vi "MES字符串.vi"(10 "MES配置输入":T2, 11 "条码字符串输入":T1) -> (2 "MES字符串":string, 3 "2~100":string)   [LabVIEW 2011]
panel:
  out "数组":string[](array[string])
  out "连接的字符串":string
  out "数组 2":string[](array[string])
  out "日期字符串":string
  out "时间字符串":string
  out "56~100":string[](array[string])
  out "已删除元素的数组子集":string[](array[string])
  out "2~55":string
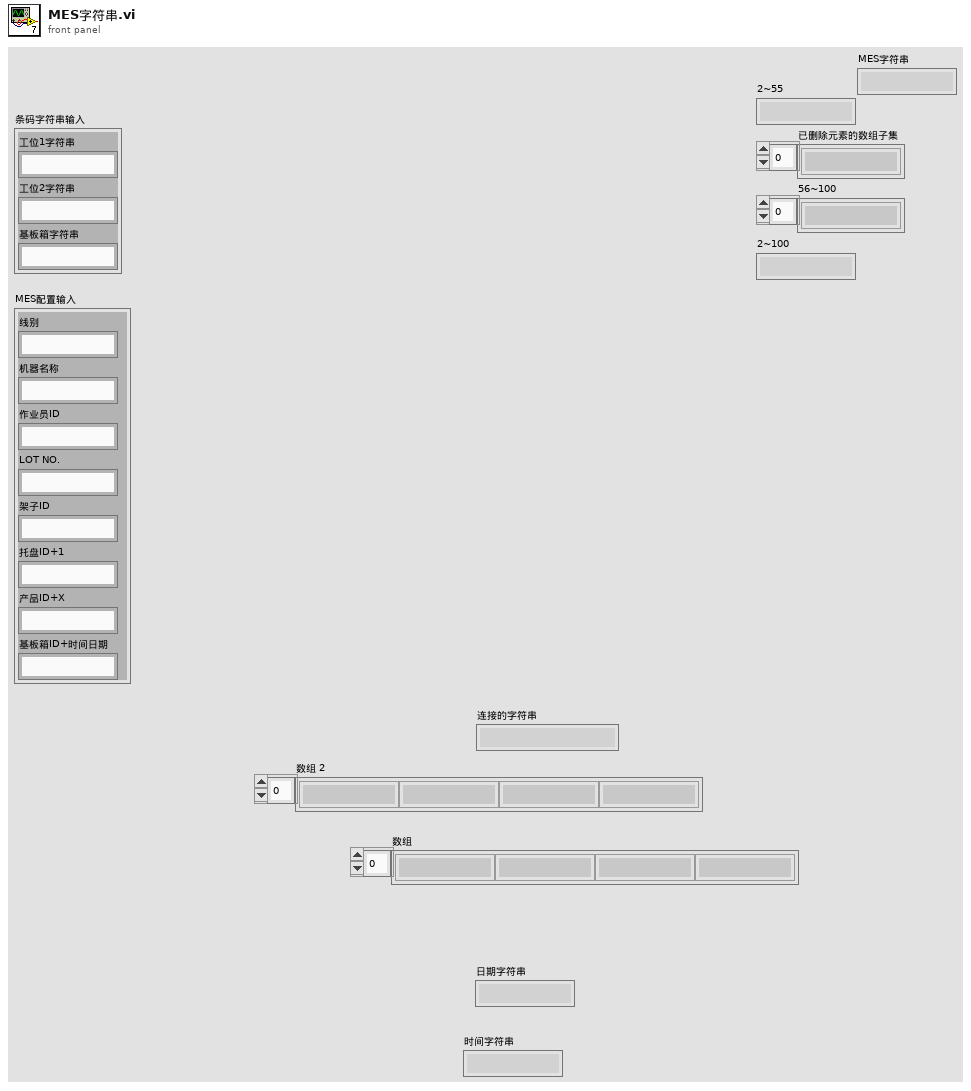
[diagram p1: front panel]
types:
  T1 = cluster{"工位1字符串":string, "工位2字符串":string, "基板箱字符串":string}
  T2 = cluster{"线别":string, "机器名称":string, "作业员ID":string, "LOT NO.":string, "架子ID":string, "托盘ID+1":string, "产品ID+X":string, "基板箱ID+时间日期":string}
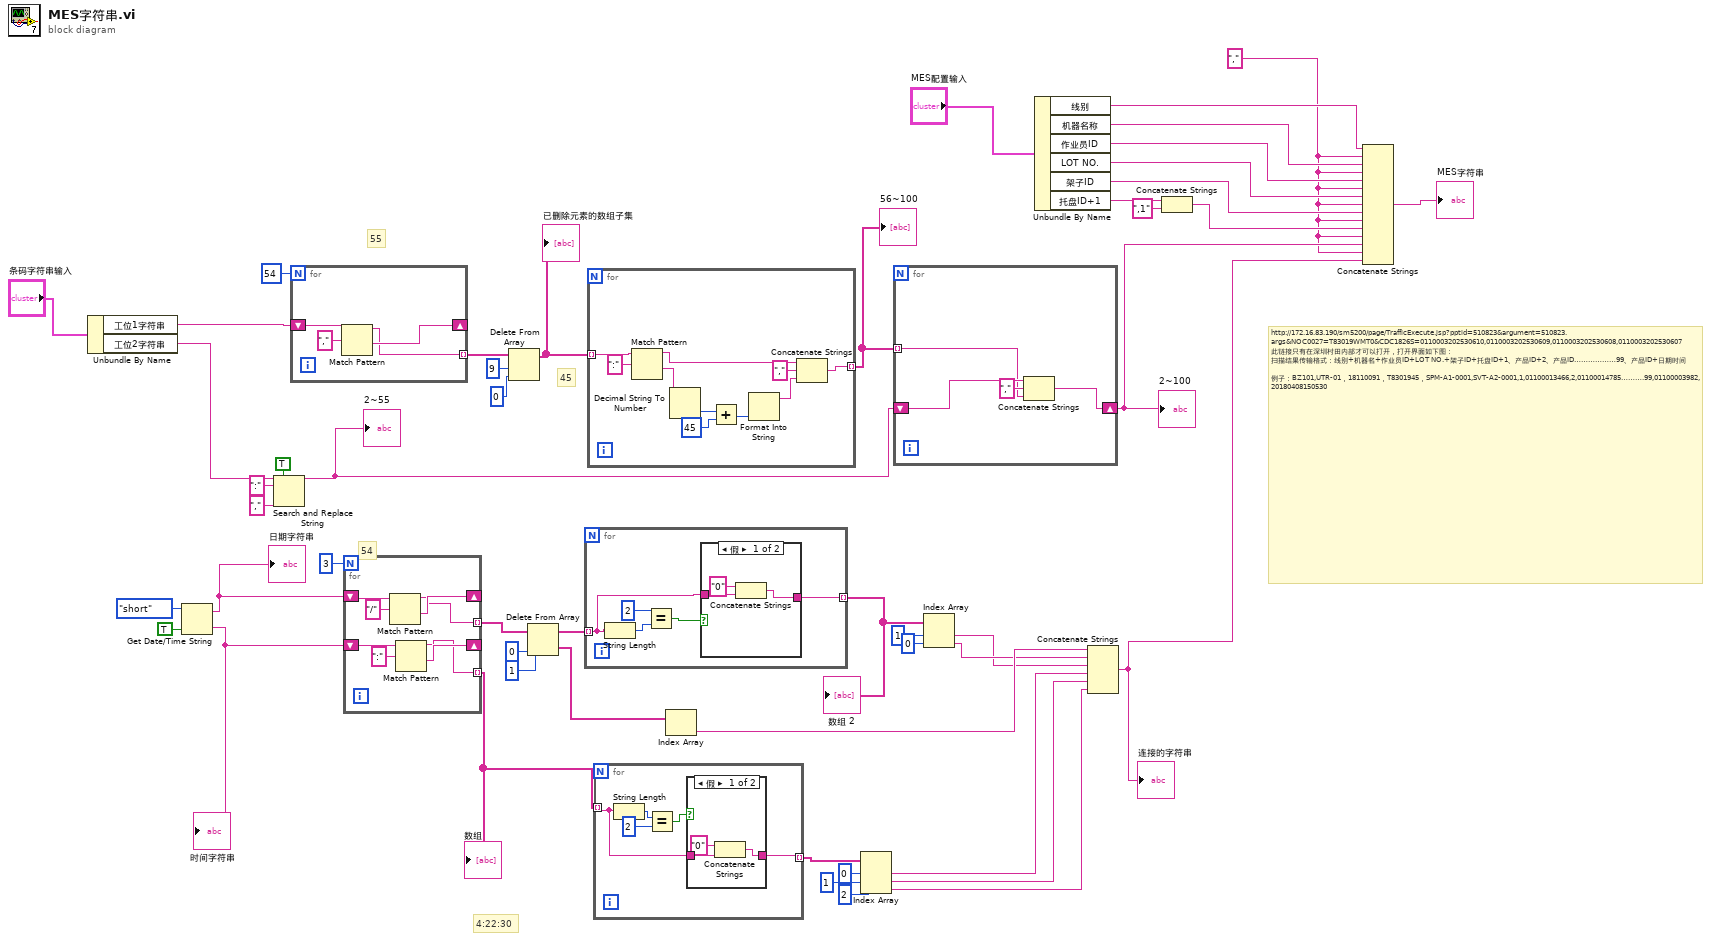
[diagram p0: block diagram]
diagram:
  w2 = ","
  # "4:22:30"
  # "http://172.16.83.190/sm5200/page/TrafficExecute.jsp?pptid=510823&argument=510823.args&NOC0027=T83019WMT0&CDC1826S=0110003202530610,0110003202530609,0110003202530608,0110003202530607\n此链接只有在深圳村田内部才可以打开，打开界面如下图：\n扫描结果传输格式：线别+机器名+作业员ID+LOT NO.+架子ID+托盘ID+1、产品ID+2、产品ID………………99、产品ID+日期时间\n                             例子：BZ101,UTR-01，18110091，T8301945，SPM-A1-0001,SVT-A2-0001,1,01100013466,2,01100014785……….99,01100003982,20180408150530"
  # "54"
  # "45"
  # "55"
  n1 = Unbundle By Name("条码字符串输入") -> ("工位1字符串"=w45:string, "工位2字符串"=w46:string)
  n2 = Get Date/Time String(date format (0)=enum16{"short", "long", "abbreviated"}."short" ("日期格式(0)"), want seconds? (F)=TRUE ("需要秒？(F)")) -> (date string=w25:string, time string=w12:string)  [unwired: 1 in]
  "时间字符串" <- w12
  "日期字符串" <- w25
  n3 = Search and Replace String(replace all?=TRUE ("替换全部？(F)"), input string=w46, search string=":" ("搜索字符串"), replace string="," ("替换字符串(\"\")")) -> (result string=w38:string)  [unwired: 4 in, 3 out]
  "2~55" <- w38
  n4 = for {
    N: 54 -> [_]
    shift-right: [w52] -> _
    shift-left: w45 -> [w54]
    tunnel: [w51] -> w43 mode=indexing
    n5 = Match Pattern(string=w54, regular expression="," ("正则表达式")) -> (before substring=w51:string, after substring=w52:string)  [unwired: 1 in, 2 out]
  }
  n6 = for {
    N: 3 -> [_]
    shift-right: [w60] -> _
    shift-left: w25 -> [w62]
    tunnel: [w59] -> w23 mode=indexing
    shift-right: [w56] -> _
    shift-left: w12 -> [w58]
    tunnel: [w55] -> w11 mode=indexing
    n7 = Match Pattern(string=w62, regular expression="/" ("正则表达式")) -> (before substring=w59:string, after substring=w60:string)  [unwired: 1 in, 2 out]
    n8 = Match Pattern(string=w58, regular expression=":" ("正则表达式")) -> (before substring=w55:string, after substring=w56:string)  [unwired: 1 in, 2 out]
  }
  "数组" <- w11
  n9 = Delete From Array(array=w43, length=9 ("长度"), index=0 ("索引")) -> (array with subset deleted=w40:string[])  [unwired: 1 out]
  "已删除元素的数组子集" <- w40
  n10 = Delete From Array(array=w23, length=1 ("长度"), index=0 ("索引")) -> (deleted portion=w19:string[], array with subset deleted=w20:string[])
  n11 = for {
    tunnel: w20 -> [w64] mode=indexing
    tunnel: [w63] -> w18 mode=indexing
    n12 = String Length(string=w64) -> (length=w67:i32)
    n13 = Equal?(x=2, y=w67) -> (x = y?=w65:bool)
    n14 = case shown="假" w65 {
      tunnel: w64 -> [w70 w71]
      tunnel: [w68 w71] -> w63
      frame False {
        n15 = Concatenate Strings("0" ("字符串"), w70) -> (w68:string)
      }
      frame True {
      }
    }
  }
  "数组 2" <- w18
  n16 = for {
    tunnel: w40 -> [w81] mode=indexing
    tunnel: [w74] -> w39 mode=indexing
    n17 = Match Pattern(string=w81, regular expression=":" ("正则表达式")) -> (before substring=w79:string, after substring=w78:string)  [unwired: 1 in, 2 out]
    n18 = Decimal String To Number(string=w78) -> (number=w77:i32)  [unwired: 2 in, 1 out]
    n19 = Add(x=w77, y=45) -> (x+y=w75:i32)
    n20 = Format Into String(w75) -> (resulting string=w73:string)  [unwired: 3 in, 1 out]
    n21 = Concatenate Strings(w79, "," ("字符串"), w73) -> (w74:string)
  }
  "56~100" <- w39
  n22 = for {
    tunnel: w11 -> [w83] mode=indexing
    tunnel: [w82] -> w10 mode=indexing
    n23 = String Length(string=w83) -> (length=w86:i32)
    n24 = Equal?(x=w86, y=2) -> (x = y?=w84:bool)
    n25 = case shown="假" w84 {
      tunnel: w83 -> [w89 w90]
      tunnel: [w88 w90] -> w82
      frame False {
        n26 = Concatenate Strings("0" ("字符串"), w89) -> (w88:string)
      }
      frame True {
      }
    }
  }
  n27 = Index Array(array=w19) -> (element=w15:string)  [unwired: 1 in]
  n28 = Index Array(array=w10, index #1=0 ("索引"), index #2=1 ("索引"), index #3=2 ("索引")) -> (element #1=w6:string, element #2=w5:string, element #3=w4:string)
  n29 = for {
    tunnel: w39 -> [w91] mode=indexing
    shift-right: [w94] -> w28
    shift-left: w38 -> [w92]
    n30 = Concatenate Strings(w92, "," ("字符串"), w91) -> (w94:string)
  }
  "2~100" <- w28
  n31 = Index Array(array=w18, index #1=1 ("索引"), index #2=0 ("索引")) -> (element #1=w13:string, element #2=w14:string)
  n32 = Unbundle By Name("MES配置输入") -> ("线别"=w36:string, "机器名称"=w33:string, "作业员ID"=w32:string, "LOT NO."=w31:string, "架子ID"=w30:string, "托盘ID+1"=w35:string)
  n33 = Concatenate Strings(w15, w14, w13, w6, w5, w4) -> (w1:string)
  "连接的字符串" <- w1
  n34 = Concatenate Strings(w35, ",1" ("字符串")) -> (w29:string)
  n35 = Concatenate Strings(w36, w2, w33, w2, w32, w2, w31, w2, w30, w2, w29, w2, w28, w2, w1) -> (→"MES字符串":string)
